vi "国弘第一点校准指令.vi"(7 "探头":T1(ring)=enum."ORP", 8 "error in (no error)":errorcluster caption="错误输入（无错误）", 10 "标准值":sgl, 11 "MB session in":refnum<class "MB_Master.lvclass">) -> (0 "error out":errorcluster caption="错误输出", 3 "MB session out":refnum<class "MB_Master.lvclass">)   [LabVIEW 2016, in "斯坦道多参数.lvlib"]
uses:
  <vilib>/Plasmionique/MB Master/MB_Master/MB_Master.lvclass
  <vilib>/Plasmionique/MB Master/MB Master.lvlib
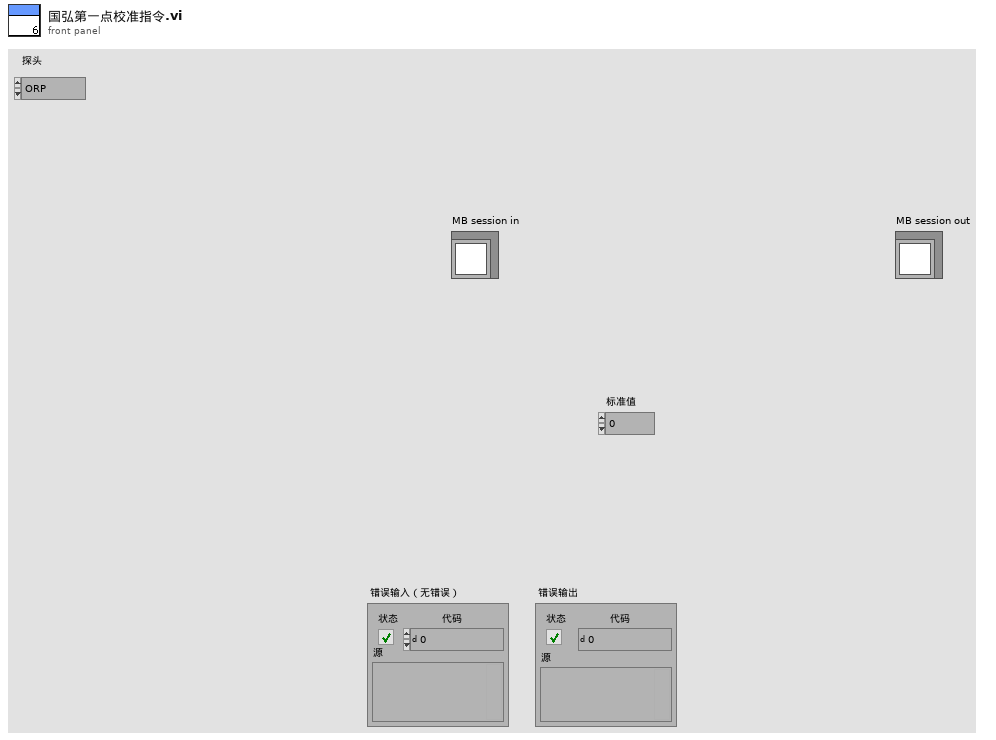
[diagram p1: front panel]
types:
  T1 = enum16{"NULL", "pH", "Cond", "DO", "Turb", "ORP"}
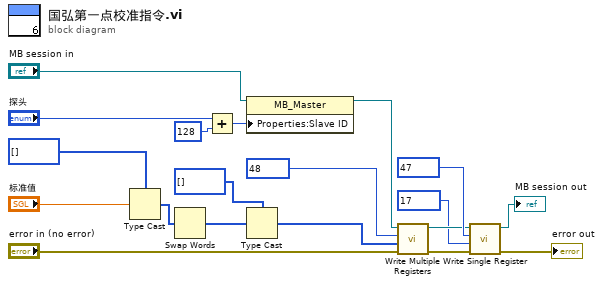
[diagram p0: block diagram]
diagram:
  n1 = Type Cast(type=u32[] [] ("数组 2"), x="标准值") -> (*(type *) &x=w13:u32[])
  n2 = Swap Words(1:w13) -> (0:w11:u32[])
  n3 = Add(x="探头", y=u16 128) -> (x+y=w17:u16)
  n4 = property class="MB_Master"(reference="MB session in", "Properties:Slave ID"=w17) -> (reference out=w15:refnum<class "MB_Master.lvclass">)  [unwired: 1 in, 1 out]
  n5 = Type Cast(type=u16[] [] ("数组 2"), x=w11) -> (*(type *) &x=w9:u16[])
  n6 = call <vilib>:"Write Multiple Registers.vi"("error in (no error)"="error in (no error)", "values"=w9, "starting address"=u16 48, "MB session in"=w15) -> ("error out"=w2:errorcluster, "MB session out"=w5:refnum<class "MB_Master.lvclass">)  [unwired: 6 in]
  n7 = call <vilib>:"Write Single Register.vi"("error in (no error)"=w2, "value"=u16 17 ("starting address"), "address"=u16 47 ("starting address"), "MB session in"=w5) -> ("error out"=→"error out":errorcluster, "MB session out"=→"MB session out":refnum<class "MB_Master.lvclass">)  [unwired: 6 in]
